vi "Decode PicoHarp TTT Data.vi"(8 "oflcorr_in":u64, 11 "rawbits":u32) -> (0 "oflcorr_out":u64, 1 "channel":u8, 2 "dtime":u32, 3 "truetime":u64, 4 "markercode":u32)   [LabVIEW 2021, in "PTU Files.lvlib"]
uses:
  PTU Files.lvlib
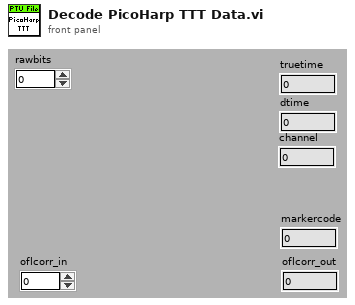
[diagram p1: front panel]
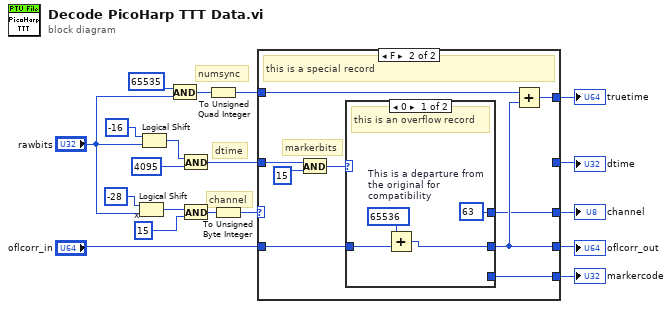
[diagram p0: block diagram]
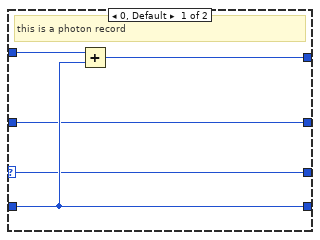
[diagram p2: hidden frame]
diagram:
  w4 = u32 15  # x
  # "dtime"
  # "channel"
  # "numsync"
  n1 = Logical Shift(y=-28, x="rawbits") -> (x << y=w12:u32)
  n2 = Logical Shift(y=-16, x="rawbits") -> (x << y=w15:u32)
  n3 = And(x=u32 65535, y="rawbits") -> (x .and. y?=w17:u32)
  n4 = And(x=w15, y=u32 4095 ("x")) -> (x .and. y?=w13:u32)
  n5 = And(x=w12, y=w4) -> (x .and. y?=w5:u32)
  n6 = To Unsigned Quad Integer(1:w17) -> (0:w2:u64)
  n7 = To Unsigned Byte Integer(number=w5) -> (unsigned 8bit integer=w1:u8)
  n8 = case shown="F" w1 {
    selector: w1 -> [w21 _]
    tunnel: w2 -> [w20 w28]
    tunnel: "oflcorr_in" -> [w24 w31]
    tunnel: [w24 w29] -> w9
    tunnel: w13 -> [w22 w32]
    tunnel: [w23 w30] -> w7
    tunnel: [w22 _] -> w6
    tunnel: [w21 w26] -> w8
    tunnel: [_ w25] -> w3
    frame 0, Default {
      # "this is a photon record"
      n9 = Add(x=w20, y=w24) -> (x+y=w23:u64)
    }
    frame 15 {
      # "markerbits"
      # "this is a special record"
      n10 = And(x=w32, y=u32 15 ("x")) -> (x .and. y?=w27:u32)
      n11 = case shown="0" w27 {
        selector: w27 -> [_ w38]
        tunnel: w31 -> [w37 w39]
        tunnel: [w36 w39] -> w29
        tunnel: [w34 _] -> w26
        tunnel: [_ w38] -> w25
        frame 0 {
          w34 = u8 63  # This is a departure from the original for compatibility
          # "this is an overflow record"
          n12 = Add(x=u64 65536, y=w37) -> (x+y=w36:u64)
        }
        frame 1, Default {
          # "this is a marker record"
        }
      }
      n13 = Add(x=w28, y=w29) -> (x+y=w30:u64)
    }
  }
  "channel" <- w8
  "truetime" <- w7
  "markercode" <- w3
  "oflcorr_out" <- w9
  "dtime" <- w6
